vi "Update Pump State.vi"(6 "Sender":refnum<class "Sender.lvclass">, 10 "Pump State":bool, 11 "Update Pump State in":refnum<class "Update Pump State.lvclass">) -> (0 "Error out":errorcluster, 3 "Update Pump State out":refnum<class "Update Pump State.lvclass">)   [LabVIEW 2025, in "Update Pump State Msg.lvlib" / "Update Pump State.lvclass"]
uses:
  Update Pump State.lvclass
  <vilib>/Nathan Davis/jettl/jettl/jettl/Sender/Sender/Sender.lvclass
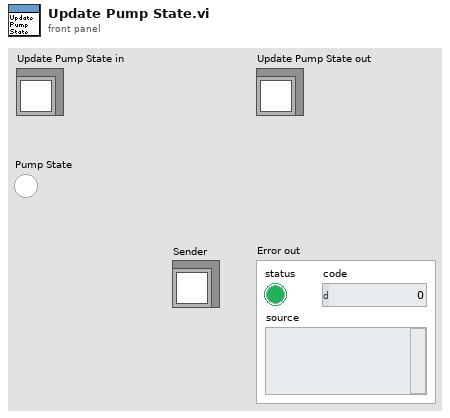
[diagram p1: front panel]
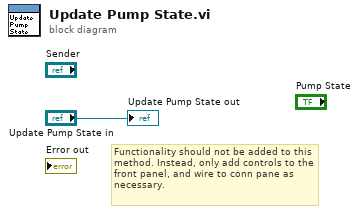
[diagram p0: block diagram]
diagram:
  # "Functionality should not be added to this method. Instead, only add controls to the front panel, and wire to conn pane as necessary."
  "Update Pump State out" <- "Update Pump State in"
